vi "Weather_Queues.vi"() -> ()   [LabVIEW 2013]
panel:
  out "Weather Queues":T1
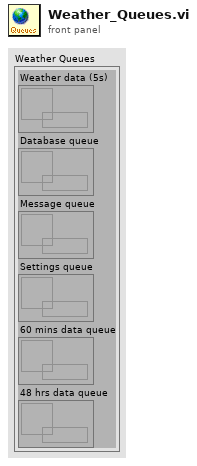
[diagram p1: front panel]
types:
  T1 = cluster{"Weather data (5s)":refnum<queue>, "Database queue":refnum<queue>, "Message queue":refnum<queue>, "Settings queue":refnum<queue>, "60 mins data queue":refnum<queue>, "48 hrs data queue":refnum<queue>}
diagram:
